vi "ProgramaticallyRunSequenceOnLogin.vi"(7 "Mode":enum16{"Initialize", "Run"}(ring)=enum."Run", 8 "error in (no error)":errorcluster, 9 "Visible Controls.Entry Point 1 Button":refnum<k7>, 10 "Visible Controls.TestStand UI Label Control":refnum<k7>, 11 "Manager Controls.Application Manager":refnum<k7>) -> (0 "error out":errorcluster, 3 "wasSetup":bool)   [LabVIEW 2015]
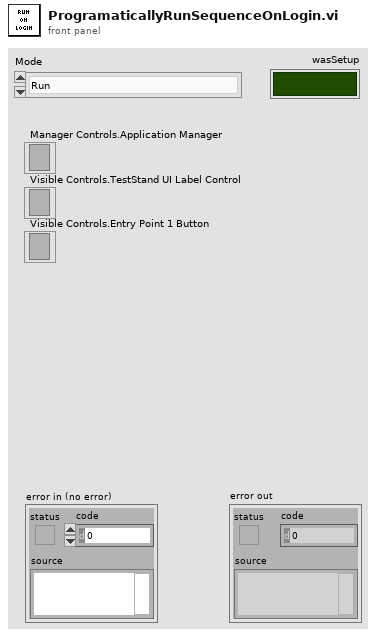
[diagram p1: front panel]
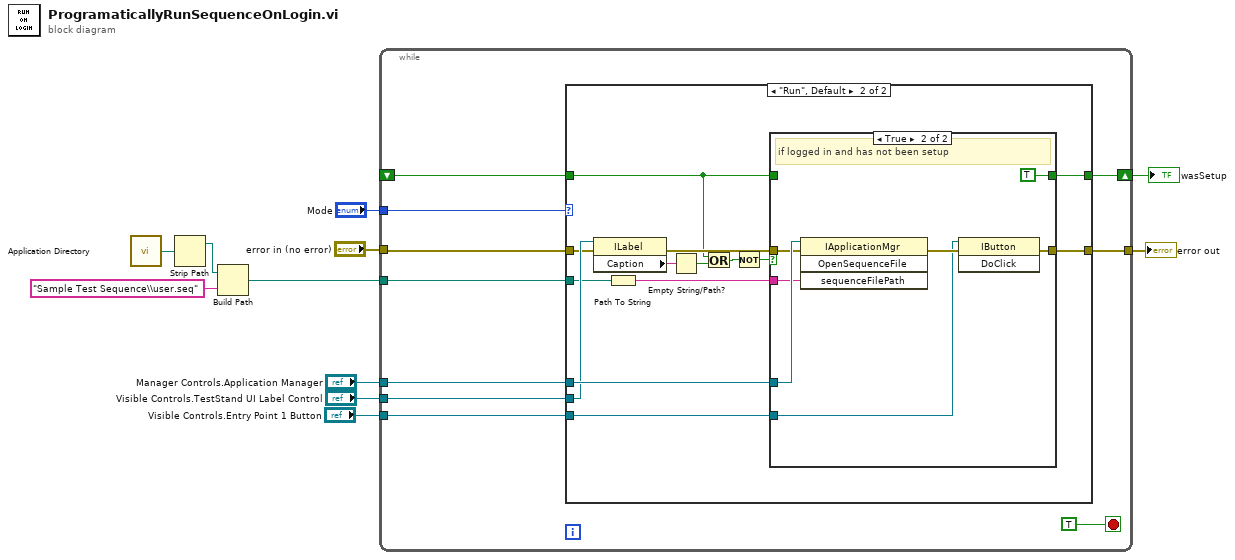
[diagram p0: block diagram]
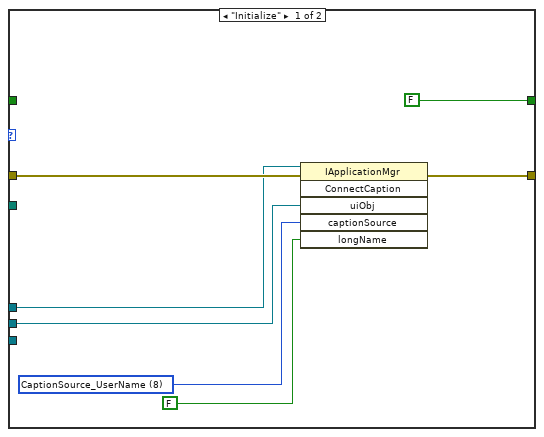
[diagram p2: hidden frame]
diagram:
  n1 = call <vilib>:"Application Directory.vi"() -> ("Application Directory"=w4:path)
  n2 = Strip Path(path=w4) -> (stripped path=w3:path)  [unwired: 1 out]
  n3 = Build Path(base path=w3, name or relative path="Sample Test Sequence\\user.seq") -> (appended path=w1:path)
  n4 = while {
    tunnel: "Mode" -> [w21]
    shift-right: [w19] -> w5
    shift-left: _ -> [w18]
    tunnel: w1 -> [w17]
    tunnel: "error in (no error)" -> [w16]
    tunnel: [w15] -> w9
    tunnel: "Manager Controls.Application Manager" -> [w14]
    tunnel: "Visible Controls.TestStand UI Label Control" -> [w13]
    tunnel: "Visible Controls.Entry Point 1 Button" -> [w12]
    stop <- TRUE stop-if-true
    n5 = case shown="\"Run\", Default" w21 {
      tunnel: [FALSE w34] -> w19
      tunnel: w18 -> [_ w32]
      tunnel: w17 -> [_ w37]
      tunnel: w16 -> [w25 w39]
      tunnel: [w24 w42] -> w15
      tunnel: w14 -> [w23 w41]
      tunnel: w13 -> [w22 w40]
      tunnel: w12 -> [_ w29]
      frame "Initialize" {
        w27 = 8 items=["CaptionSource_NotASource", "CaptionSource_MacroExpression", "CaptionSource_UUTSerialNumber", "CaptionSource_UUTStatus", "CaptionSource_BatchSerialNumber", "CaptionSource_BatchStatus", "CaptionSource_BatchState", "CaptionSource_ModelState", "CaptionSource_UserName", "CaptionSource_ProgressText", "CaptionSource_ProgressPercent", "CaptionSource_CurrentSequenceFile", "CaptionSource_CurrentSequenceFileComment", "CaptionSource_CurrentSequence", "CaptionSource_CurrentSequenceComment", "CaptionSource_CurrentStepGroup", "CaptionSource_CurrentStep", "CaptionSource_CurrentStepComment", "CaptionSource_CurrentStepIndex_ZeroBased", "CaptionSource_CurrentTestIndex_OneBased", "CaptionSource_SelectedSteps_ZeroBased", "CaptionSource_SelectedTests_OneBased", "CaptionSource_NumberOfSteps", "CaptionSource_NumberOfTests", "CaptionSource_CurrentExecution", "CaptionSource_CurrentThread", "CaptionSource_CurrentCallStackEntry", "CaptionSource_CurrentProcessModelFile", "CaptionSource_ReportLocation", "CaptionSource_TestSocketIndex", "CaptionSource_Time", "CaptionSource_Date", "CaptionSource_CurrentSequenceFile_WithoutFileState", "CaptionSource_CurrentSequenceFile_FileStateOnly"] ("captionSource")
        n6 = invoke class="IApplicationMgr" method="ConnectCaption"(reference=w23, error in=w25, "uiObj"=w22, "captionSource"=w27, "longName"=FALSE) -> (error out=w24:errorcluster)  [unwired: 1 in, 5 out]
      }
      frame "Run", Default {
        n7 = property class="ILabel"(reference=w40, error in=w39) -> (error out=w38:errorcluster, "Caption"=w35:string)  [unwired: 1 out]
        n8 = Path To String(path=w37) -> (string=w36:string)
        n9 = Empty String/Path?(string/path=w35) -> (empty?=w33:bool)
        n10 = Or(x=w32, y=w33) -> (x .or. y?=w31:bool)
        n11 = Not(x=w31) -> (.not. x?=w30:bool)
        n12 = case shown="True" w30 {
          tunnel: [w44 w50] -> w42
          tunnel: w41 -> [_ w49]
          tunnel: w38 -> [w44 w48]
          tunnel: w36 -> [_ w47]
          tunnel: [w43 TRUE] -> w34
          tunnel: w32 -> [w43 _]
          tunnel: w29 -> [_ w45]
          frame False {
          }
          frame True {
            # "if logged in and has not been setup"
            n13 = invoke class="IApplicationMgr" method="OpenSequenceFile"(reference=w49, error in=w48, "sequenceFilePath"=w47) -> (error out=w51:errorcluster)  [unwired: 1 in, 3 out]
            n14 = invoke class="IButton" method="DoClick"(reference=w45, error in=w51) -> (error out=w50:errorcluster)  [unwired: 1 in, 2 out]
          }
        }
      }
    }
  }
  "error out" <- w9
  "wasSetup" <- w5
